vi "UR3_Definition.vi"(1 "qs (deg)":sgl[](array[numeric])=[0.0, 0.0, 0.0, 0.0, 0.0, 0.0]) -> (0 "UR3":T1(array[cluster]))   [LabVIEW 2024]
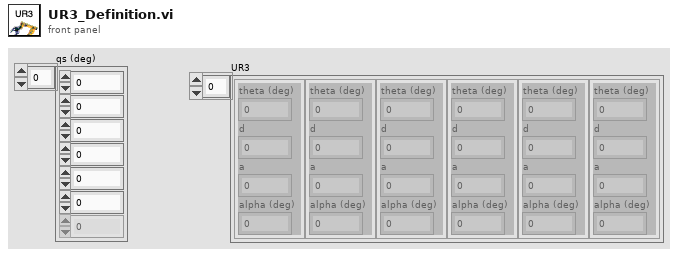
[diagram p1: front panel]
types:
  T1 = cluster{"theta (deg)":dbl, "d":dbl, "a":dbl, "alpha (deg)":dbl}[]
  T2 = cluster{"theta (deg)":dbl, "d":dbl, "a":dbl, "alpha (deg)":dbl}
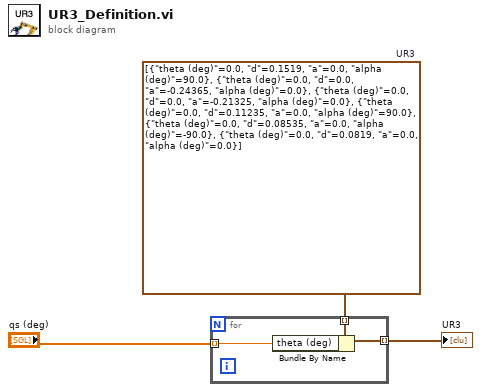
[diagram p0: block diagram]
diagram:
  w2 = T1 [{"theta (deg)"=0.0, "d"=0.1519, "a"=0.0, "alpha (deg)"=90.0}, {"theta (deg)"=0.0, "d"=0.0, "a"=-0.24365, "alpha (deg)"=0.0}, {"theta (deg)"=0.0, "d"=0.0, "a"=-0.21325, "alpha (deg)"=0.0}, {"theta (deg)"=0.0, "d"=0.11235, "a"=0.0, "alpha (deg)"=90.0}, {"theta (deg)"=0.0, "d"=0.08535, "a"=0.0, "alpha (deg)"=-90.0}, {"theta (deg)"=0.0, "d"=0.0819, "a"=0.0, "alpha (deg)"=0.0}]  # UR3
  n1 = for {
    tunnel: w2 -> [w4] mode=indexing
    tunnel: "qs (deg)" -> [w6] mode=indexing
    tunnel: [w5] -> w3 mode=indexing
    n2 = Bundle By Name(cluster=w4, "theta (deg)"=w6) -> (w5:T2)
  }
  "UR3" <- w3
